vi "GetConnectionStatistics.vi"(0 "Nav6DevRef":T1, 11 "error in (no error)":errorcluster) -> (4 "Nav6DevRef Out":T1, 6 "Update Count":i32, 8 "Byte Count":u32, 10 "IsConnected":bool, 15 "error out":errorcluster)   [LabVIEW 2013, in "Nav6.lvlib"]
uses:
  Nav6.lvlib
  Nav6DevRef.ctl
  <vilib>/Rock Robotics/WPI/SerialPort/WPI_SerialPortRef.ctl
  Nav6Mode.ctl
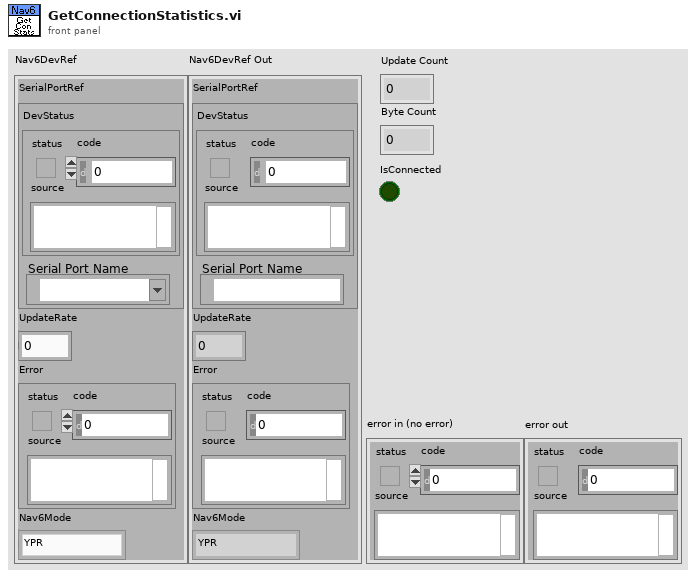
[diagram p1: front panel]
types:
  T1 = typedef "Nav6.lvlib/Nav6DevRef.ctl" = cluster{"SerialPortRef":T2, "UpdateRate":u8, "Error":errorcluster, "Nav6Mode":T3}
  T2 = typedef "WPI_SerialPortRef.ctl" = cluster{"DevStatus":errorcluster, "Serial Port Name":refnum<visa-resource-name>}
  T3 = typedef "Nav6.lvlib/Nav6Mode.ctl" = enum16{"YPR", "Gyro", "Quaternion"}
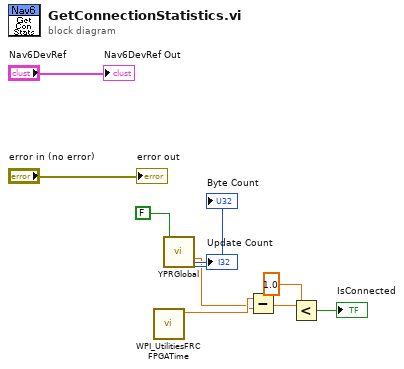
[diagram p0: block diagram]
diagram:
  n1 = call <vilib>:"WPI_UtilitiesFRC FPGATime.vi"() -> ("FPGA Time"=w5:dbl)  [unwired: 10 in, 1 out]
  n2 = call "YPRGlobal.vi"("Update"=FALSE) -> ("Last Update"=w4:dbl, "Update Count"=→"Update Count":i32, "Byte Count Out"=→"Byte Count":u32)  [unwired: 20 in, 4 out]
  n3 = Subtract(x=w5, y=w4) -> (x-y=w3:dbl)
  n4 = Less?(x=w3, y=1.0) -> (x < y?=→"IsConnected":bool)
  "Nav6DevRef Out" <- "Nav6DevRef"
  "error out" <- "error in (no error)"
